vi "3_1.vi"() -> ()   [LabVIEW 2021]
uses:
  <vilib>/Utility/miscctls.llb/LVMapReplaceAction.ctl
panel:
  out "x*y":i32
  out "number 3":fxp<+,12,12>
  out "number 2":fxp<+,12,12>
  out "value 2":i32
  out "value":i32
  out "Array 2":string[](array[string])
  out "Array":string[][](array[string])
  out "Formatted 1D String Array":string[](array[string])
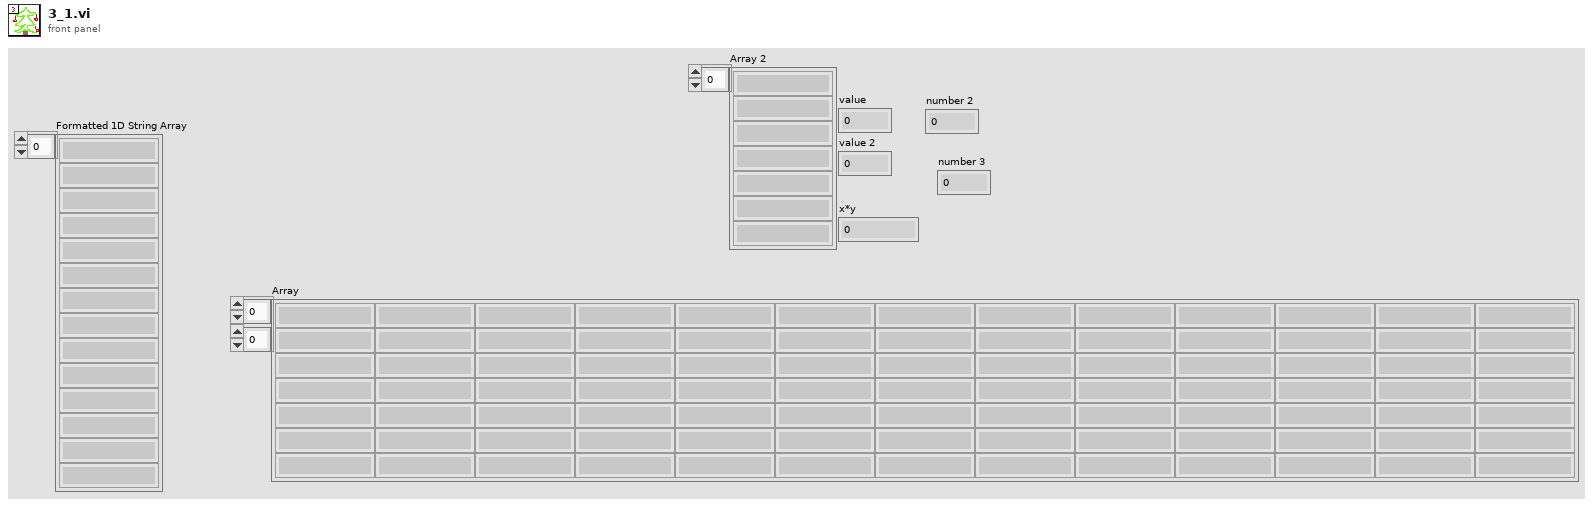
[diagram p1: front panel]
types:
  T1 = typedef "LVMapReplaceAction.ctl" = enum32{"Modify Entry only if found", "Add or Modify Entry", "Delete Entry"}
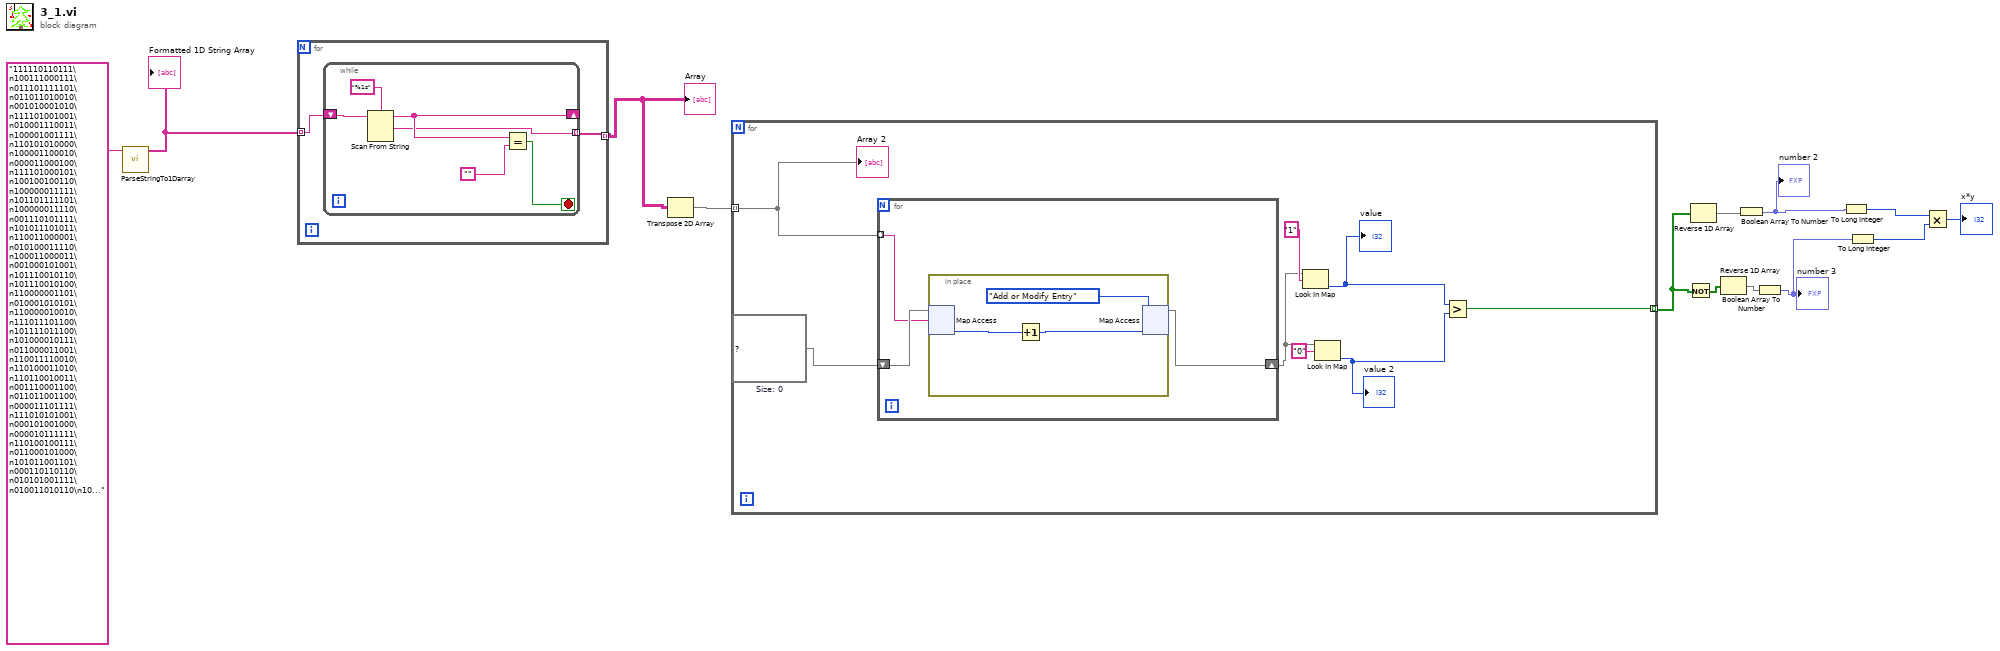
[diagram p0: block diagram]
diagram:
  n1 = call "ParseStringTo1Darray.vi"("Copied Input From Advent Of Code Website"="111110110111\n100111000111\n011101111101\n011011010010\n001010001010\n111101001001\n010001110011\n100001001111\n110101010000\n100001100010\n000011000100\n111101000101\n100100100110\n100000011111\n101101111101\n100000011110\n001110101111\n101011101011\n110011000001\n010100011110\n100011000011\n001000101001\n101110010110\n101110010100\n110000001101\n010001010101\n110000010010\n111011101100\n101111011100\n101000010111\n011000011001\n110011110010\n110100011010\n110110010011\n001110001100\n011011001100\n000011101111\n111010101001\n000101001000\n000010111111\n110100100111\n011000101000\n101011001101\n000110110110\n010101001111\n010011010110\n10..." ("String")) -> ("Formatted 1D String Array"=w12:string[])  [unwired: 10 in]
  "Formatted 1D String Array" <- w12
  n2 = for {
    tunnel: w12 -> [w15] mode=indexing
    tunnel: [w14] -> w11 mode=indexing
    n3 = while {
      shift-right: [w18] -> _
      shift-left: w15 -> [w16]
      tunnel: [w17] -> w14 mode=indexing
      stop <- w19 stop-if-true
      n4 = Scan From String(format string="%1s", input string=w16) -> (remaining string=w18:string, output 1=w17:string)  [unwired: 3 in, 2 out]
      n5 = Equal?(x=w18, y="") -> (x = y?=w19:bool)
    }
  }
  "Array" <- w11
  n6 = Transpose 2D Array(2D array=w11) -> (transposed array=w10:string[][])
  n7 = for {
    tunnel: w10 -> [w29] mode=indexing
    tunnel: [w22] -> w8 mode=indexing
    w28 = map{string, i32} {}  # Size: 0
    n8 = for {
      tunnel: w29 -> [w31] mode=indexing
      shift-right: [w30] -> w26
      shift-left: w28 -> [w32]
      n9 = in-place {
        n10 = in-place-map #1(w32, w31) -> (w35:i32)  [unwired: 1 in, 1 out]
        n11 = Increment(x=w35) -> (x+1=w34:i32)
        n12 = in-place-map #1(w34, LVMapReplaceAction."Add or Modify Entry" ("action")) -> (w30:map{string, i32})  [unwired: 2 out]
      }
    }
    n13 = Look In Map(map=w26, key="1") -> (value=w24:i32)  [unwired: 1 in, 1 out]
    "value" <- w24
    n14 = Look In Map(map=w26, key="0") -> (value=w23:i32)  [unwired: 1 in, 1 out]
    "value 2" <- w23
    n15 = Greater?(x=w24, y=w23) -> (0:w22:bool)
    "Array 2" <- w29
  }
  n16 = Not(x=w8) -> (.not. x?=w7:bool[])
  n17 = Reverse 1D Array(array=w8) -> (reversed array=w9:bool[])
  n18 = Reverse 1D Array(array=w7) -> (reversed array=w6:bool[])
  n19 = Boolean Array To Number(Boolean array=w9) -> (number=w5:fxp<+,12,12>)
  "number 2" <- w5
  n20 = Boolean Array To Number(Boolean array=w6) -> (number=w4:fxp<+,12,12>)
  "number 3" <- w4
  n21 = To Long Integer(number=w5) -> (32bit integer=w3:i32)
  n22 = To Long Integer(number=w4) -> (32bit integer=w2:i32)
  n23 = Multiply(x=w3, y=w2) -> (x*y=→"x*y":i32)
